vi "RT Apply Target Disk Image Core.vi"(4 "file blacklist":string[](array[string]), 6 "restart after imaging? (T)":bool=TRUE, 8 "error in (no error)":errorcluster, 10 "image path":path, 11 "target address":string) -> (0 "error out":errorcluster, 3 "IP settings after restart":T1)   [LabVIEW 2020, in "NI_Real-Time Libraries.lvlib"]
doc: "LabVIEW no longer supports this VI. For information about replacing the RT Utility VIs, refer to ni.com/info and enter the Info Code RT_Utility_Replace. Replaces the entire contents of the primary hard drive on the RT target with the files in the target disk image you specify.\n\n<B>target address</B> specifies the IP address or DNS name of the target. \n\n<B>image file path</B> specifies the local path of the disk image to load onto the RT target. \n\n<B>error in</B> describes error conditions that occur before this node runs. This input provides standard error in functionality. \n\n<B>restart after imaging</B> specifies whether to restart the target after applying the target disk image. If this input is FALSE, the RT target remains in install mode after this VI runs. If this input is TRUE, the RT target restarts into normal running mode.\n\n<B>file blacklist</B> specifies an array of file paths to exclude from the target image. To enable filtering through strict matching, the data type of this control is an array of strings rather than an array of paths. \n\n<B>IP settings after restart</B> returns the IP settings of the RT target. If the IP settings change upon restarting, this output returns the new IP settings that take effect after the target restarts. If the previous IP address of the target is in use by another device on the network and the target is configured to use DHCP, the IP address of the target might change upon restarting.\n\n<B>IP address</B> is the IP address of the networked device. \n\n<B>DNS name</B> is the network DNS name of the target. \n\n<B>subnet mask</B> is the bit mask used to identify the subnet in which the target resides on the network. \n\n<B>gateway</B> is the network gateway used by the target. \n\n<B>DNS server</B> is the domain name server used by the target. \n\n<B>error out</B> contains error information. This output provides standard error out functionality. \n\n\nRT Apply Target Disk Image Details\nIf you need to perform additional configuration operations, set <B>restart after imaging?</B> to FALSE. When <B>restart after imaging?</B> is FALSE, <B>IP settings after restart</B> returns an empty cluster. When <B>restart after imaging?</B> is TRUE, this VI waits to finish until the real-time operating system has started and can communicate over the network. However, because the RT target requires additional time to load LabVIEW, drivers, and startup applications, you might need to allow additional time before using the target. To avoid IP conflicts, this VI attempts to preserve the existing IP settings of the target.\n\nThis VI does not support the following use cases. Disk images based on RT targets with multiple operating systems or multiple hard disk partitions. Disk images created using an RT Desktop PC Utility USB drive. Disk images created from a target with a model code different from the model code of the target at <B>target address</B>."
uses:
  <vilib>/real-time/NI_Real-Time Libraries.lvlib
  <vilib>/real-time/rtutility.llb/subVIs/IP Settings.ctl
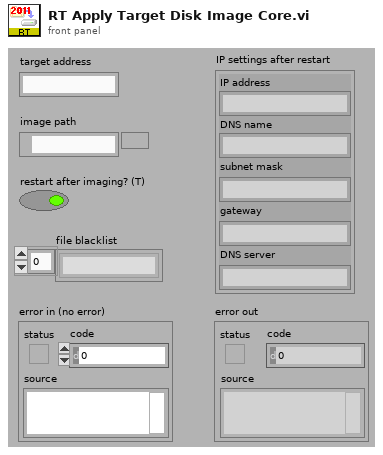
[diagram p1: front panel]
types:
  T1 = typedef "NI_Real-Time Libraries.lvlib/IP Settings.ctl" = cluster{"IP address":string, "DNS name":string, "subnet mask":string, "gateway":string, "DNS server":string}
  T2 = cluster{"local subnet?":bool, "IP address":string}
  T3 = typedef "NI_Real-Time Libraries.lvlib/RT Target Information.ctl" = cluster{"IP settings":T1, "MAC address":string, "serial number":u32, "system state":string, "model name":string, "model code":string, "password protected restarts?":bool, "halt if TCP/IP fails?":bool, "locked?":bool, "use DHCP?":bool}
  T4 = typedef "NI_FTP.lvlib/FTP Session.ctl" = refnum<k5>
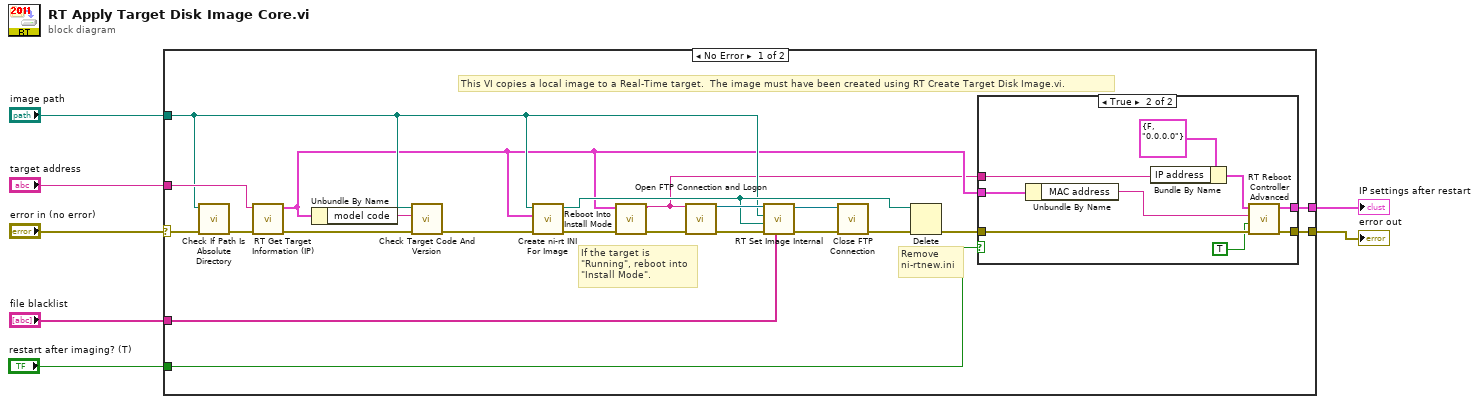
[diagram p0: block diagram]
diagram:
  n1 = case shown="No Error" "error in (no error)" {
    selector: "error in (no error)" -> [w13 w40]
    tunnel: [w28 w40] -> w7
    tunnel: "image path" -> [w10 _]
    tunnel: [w29 _] -> w5
    tunnel: "file blacklist" -> [w18 _]
    tunnel: "restart after imaging? (T)" -> [w24 _]
    tunnel: "target address" -> [w11 _]
    frame No Error {
      # "If the target is \"Running\", reboot into \"Install Mode\"."
      # "This VI copies a local image to a Real-Time target.  The image must have been created using RT Create Target Disk Image.vi."
      # "Remove \nni-rtnew.ini"
      n2 = call <vilib>:"Check If Path Is Absolute Directory.vi"("error in (no error)"=w13, "path"=w10) -> ("error out"=w14:errorcluster)  [unwired: 9 out]
      n3 = call <vilib>:"RT Get Target Information (IP).vi"("error in (no error)"=w14, "target address"=w11) -> ("error out"=w12:errorcluster, "target information"=w9:T3)  [unwired: 1 in, 7 out]
      n4 = Unbundle By Name(w9) -> ("model code"=w26:string)
      n5 = call <vilib>:"Check Target Code And Version.vi"("error in (no error)"=w12, "destination target code"=w26, "image path"=w10) -> ("error out"=w25:errorcluster)  [unwired: 8 out]
      n6 = call <vilib>:"Create ni-rt INI For Image.vi"("error in (no error)"=w25, "RT target information"=w9, "image path"=w10) -> ("error out"=w15:errorcluster, "tmp ni-rt path"=w17:path)  [unwired: 7 out]
      n7 = call <vilib>:"Reboot Into Install Mode.vi"("error in (no error)"=w15, "RT target information"=w9) -> ("error out"=w16:errorcluster, "IP address"=w8:string)  [unwired: 8 out]
      n8 = call <vilib>:"Open FTP Connection and Logon.vi"("address"=w8, "error in (no error)"=w16) -> ("ftp session out"=w22:T4, "error out"=w21:errorcluster)  [unwired: 3 in, 9 out]
      n9 = call <vilib>:"RT Set Image Internal.vi"("blacklist file paths"=w18, "error in (no error)"=w21, "new ini path"=w17, "local image path"=w10, "ftp session"=w22) -> ("error out"=w19:errorcluster, "ftp session out"=w20:T4)  [unwired: 5 out]
      n10 = call <vilib>:"Close FTP Connection.vi"("error in (no error)"=w19, "ftp session"=w20) -> ("error out"=w23:errorcluster)  [unwired: 9 out]
      n11 = Delete(path (use dialog)=w17, error in=w23) -> (error out=w27:errorcluster)  [unwired: 5 out]
      n12 = case shown="True" w24 {
        tunnel: [_ w39] -> w29
        tunnel: [w30 w38] -> w28
        tunnel: w27 -> [w30 w37]
        tunnel: w9 -> [_ w34]
        tunnel: w8 -> [_ w31]
        frame False {
        }
        frame True {
          n13 = Unbundle By Name(w34) -> ("MAC address"=w33:string)
          n14 = Bundle By Name(cluster=T2 {"local subnet?"=FALSE, "IP address"="0.0.0.0"} ("system location (local subnet)"), "IP address"=w31) -> (w32:T2)
          n15 = call <vilib>:"RT Reboot Controller Advanced.vi"("error in (no error)"=w37, "Wait for reboot? (F)"=TRUE ("Install Mode"), "MAC address"=w33, "system location (local subnet)"=w32) -> ("error out"=w38:errorcluster, "IP settings after reboot"=w39:T1)  [unwired: 6 out]
        }
      }
    }
    frame Error {
    }
  }
  "error out" <- w7
  "IP settings after restart" <- w5
